vi "Create Notifiers.vi"(8 "error in (no error)":errorcluster) -> (0 "error out":errorcluster, 3 "output cluster":T1)   [LabVIEW 2015]
uses:
  Notifier.ctl
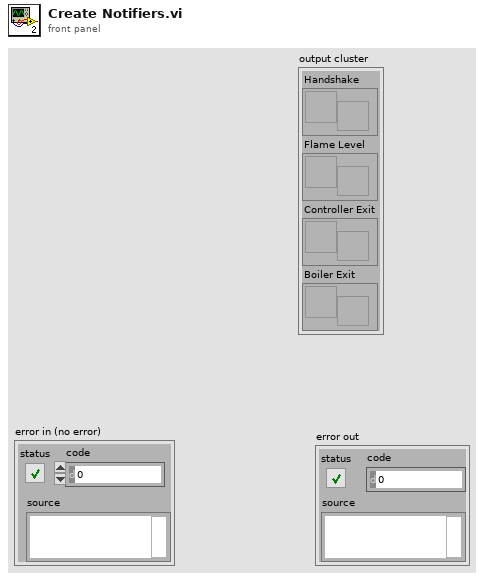
[diagram p1: front panel]
types:
  T1 = typedef "Notifier.ctl" = cluster{"Handshake":refnum<notifier>, "Flame Level":refnum<notifier>, "Controller Exit":refnum<notifier>, "Boiler Exit":refnum<notifier>}
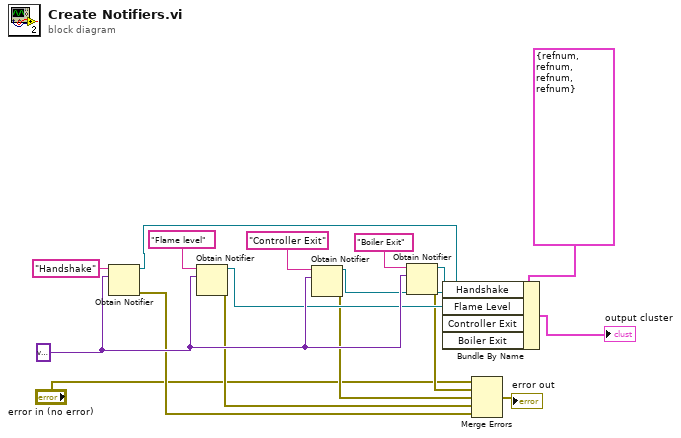
[diagram p0: block diagram]
diagram:
  w14 = variant
  n1 = Obtain Notifier(name (unnamed)="Handshake", notification data type=w14) -> (notifier out=w13:refnum<notifier>, error out=w6:errorcluster)  [unwired: 2 in, 1 out]
  n2 = Obtain Notifier(name (unnamed)="Flame level", notification data type=w14) -> (notifier out=w12:refnum<notifier>, error out=w7:errorcluster)  [unwired: 2 in, 1 out]
  n3 = Obtain Notifier(name (unnamed)="Controller Exit", notification data type=w14) -> (notifier out=w11:refnum<notifier>, error out=w8:errorcluster)  [unwired: 2 in, 1 out]
  n4 = Obtain Notifier(name (unnamed)="Boiler Exit", notification data type=w14) -> (notifier out=w10:refnum<notifier>, error out=w9:errorcluster)  [unwired: 2 in, 1 out]
  n5 = Bundle By Name(cluster=T1 {"Handshake"=refnum, "Flame Level"=refnum, "Controller Exit"=refnum, "Boiler Exit"=refnum}, "Handshake"=w13, "Flame Level"=w12, "Controller Exit"=w11, "Boiler Exit"=w10) -> (→"output cluster":T1)
  n6 = Merge Errors("error in (no error)", w9, w8, w7, w6) -> (→"error out":errorcluster)
